vi "setBlockStatistics.vi"(1 "Raw Signals":dbl[][](array[numeric]), 2 "PostProDataPerBlock in":T1[][](array[typedef]), 3 "Channel Names":string[](array[string])) -> (0 "PostProDataPerBlock out":T1[][](array[typedef]))   [LabVIEW 2013]
uses:
  Controls/postProData.ctl
  Controls/U.ctl
  Globals/measurementGlobal.vi
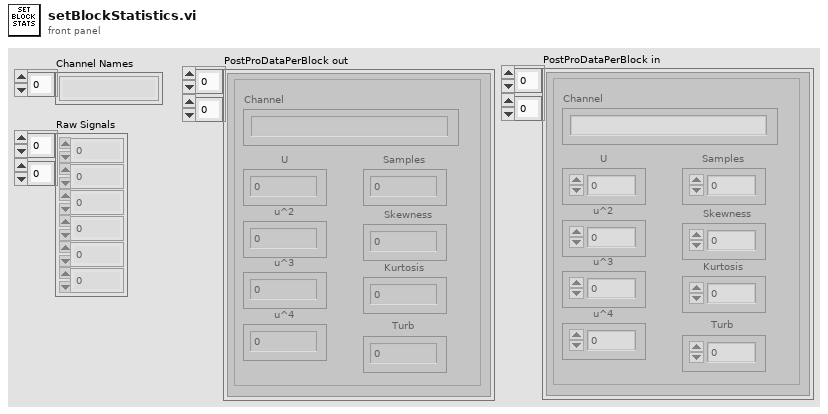
[diagram p1: front panel]
types:
  T1 = typedef "postProData.ctl" = cluster{"Channel":string, "Samples":i32, "U":dbl, "u^2":dbl, "u^3":dbl, "u^4":dbl, "Kurtosis":dbl, "Skewness":dbl, "Turb":dbl}
  T2 = typedef "U.ctl" = cluster{"Samples":dbl, "U":dbl, "U2":dbl, "U3":dbl, "U4":dbl}
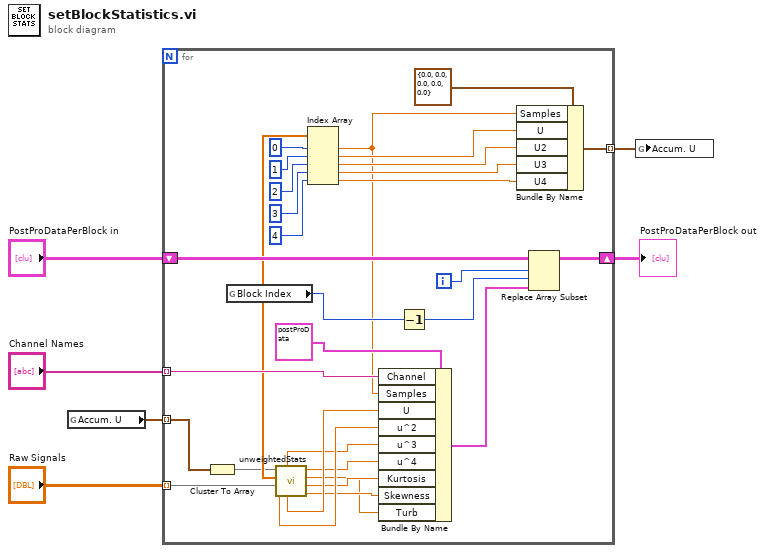
[diagram p0: block diagram]
diagram:
  n1 = global read "measurementGlobal.vi" "Accum. U"() -> (w1:T2[])
  n2 = for {
    tunnel: "Raw Signals" -> [w29] mode=indexing
    tunnel: "Channel Names" -> [w34] mode=indexing
    shift-right: [w37] -> w6
    shift-left: "PostProDataPerBlock in" -> [w36]
    tunnel: [w10] -> w2 mode=indexing
    tunnel: w1 -> [w9] mode=indexing
    i -> [w32]
    n3 = Cluster To Array(cluster=w9) -> (array=w8:dbl[])
    n4 = global read "measurementGlobal.vi" "Block Index"() -> (w31:i32)
    n5 = call "unweightedStats.vi"("U"=w29, "Data Shift Input"=w8) -> ("Skew"=w26:dbl, "Kurt"=w25:dbl, "u'/U"=w24:dbl, "u^4"=w23:dbl, "U"=w28:dbl, "u^3"=w22:dbl, "u^2"=w27:dbl, "Data Shift Output"=w20:dbl[])
    n6 = Index Array(array=w20, index #1=0 ("index"), index #2=1 ("index"), index #3=2 ("index"), index #4=3 ("index"), index #5=4 ("index")) -> (element #1=w7:dbl, element #2=w14:dbl, element #3=w13:dbl, element #4=w12:dbl, element #5=w11:dbl)
    n7 = Bundle By Name(cluster=T1 {"Channel"="", "Samples"=0, "U"=0.0, "u^2"=0.0, "u^3"=0.0, "u^4"=0.0, "Kurtosis"=0.0, "Skewness"=0.0, "Turb"=0.0} ("Post Pro Data"), "Channel"=w34, "Samples"=w7, "U"=w28, "u^2"=w27, "u^3"=w22, "u^4"=w23, "Kurtosis"=w25, "Skewness"=w26, "Turb"=w24) -> (w33:T1)
    n8 = Decrement(x=w31) -> (x-1=w30:i32)
    n9 = Bundle By Name(cluster=T2 {"Samples"=0.0, "U"=0.0, "U2"=0.0, "U3"=0.0, "U4"=0.0} ("Accum. U"), "Samples"=w7, "U"=w14, "U2"=w13, "U3"=w12, "U4"=w11) -> (w10:T2)
    n10 = Replace Array Subset(array=w36, new element=w33, index (row)=w32, index (col)=w30) -> (w37:T1[][])
  }
  "PostProDataPerBlock out" <- w6
  n11 = global write "measurementGlobal.vi" "Accum. U"(w2) -> ()
